vi "svc_Increment Histogram and Count.vi"(7 "counts in":T1, 10 "bin index":i32, 11 "histogram in":u64[](array[numeric])) -> (3 "histogram out":u64[](array[numeric]), 5 "counts out":T1)   [LabVIEW 2017]
uses:
  <vilib>/addons/_NISVFA/_Shared subVIs/Controls/svc_Histogram Counts.ctl
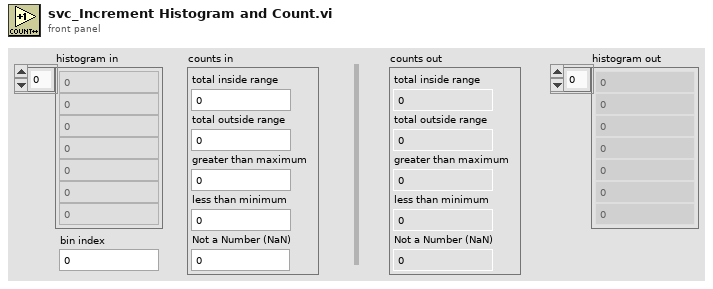
[diagram p1: front panel]
types:
  T1 = typedef "svc_Histogram Counts.ctl" = cluster{"total inside range":u64, "total outside range":u64, "greater than maximum":u64, "less than minimum":u64, "Not a Number (NaN)":u64}
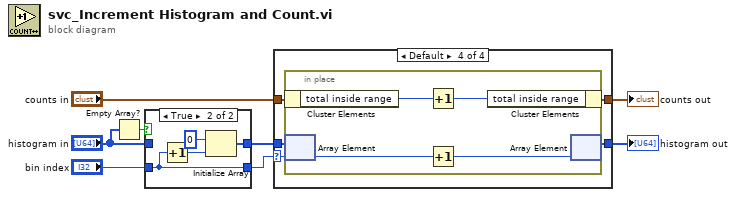
[diagram p0: block diagram]
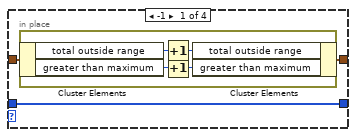
[diagram p3: hidden frame]
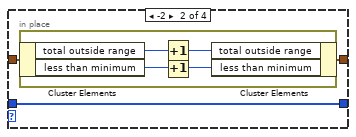
[diagram p4: hidden frame]
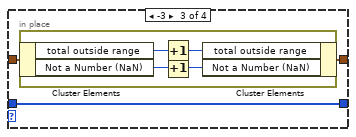
[diagram p5: hidden frame]
diagram:
  n1 = Empty Array?(array="histogram in") -> (empty?=w5:bool)
  n2 = case shown="True" w5 {
    tunnel: "histogram in" -> [w10 _]
    tunnel: "bin index" -> [w9 w11]
    tunnel: [w10 w12] -> w2
    tunnel: [w9 w11] -> w1
    frame False {
    }
    frame True {
      n3 = Increment(x=w11) -> (x+1=w14:i32)
      n4 = Initialize Array(u64 0 ("element"), w14) -> (w12:u64[])
    }
  }
  n5 = case shown="Default" w1 {
    selector: w1 -> [_ _ _ w39]
    tunnel: w2 -> [w15 w22 w31 w40]
    tunnel: [w16 w23 w29 w36] -> w6
    tunnel: "counts in" -> [w17 w24 w30 w37]
    tunnel: [w15 w22 w31 w38] -> w8
    frame -1 {
      n6 = in-place {
        n7 = in-place-cluster #1(w17) -> ("total outside range"=w21:u64, "greater than maximum"=w19:u64)
        n8 = Increment(x=w21) -> (x+1=w20:u64)
        n9 = Increment(x=w19) -> (x+1=w18:u64)
        n10 = in-place-cluster #1("total outside range"=w20, "greater than maximum"=w18) -> (w16:T1)
      }
    }
    frame -2 {
      n11 = in-place {
        n12 = in-place-cluster #2(w24) -> ("total outside range"=w28:u64, "less than minimum"=w26:u64)
        n13 = Increment(x=w28) -> (x+1=w27:u64)
        n14 = Increment(x=w26) -> (x+1=w25:u64)
        n15 = in-place-cluster #2("total outside range"=w27, "less than minimum"=w25) -> (w23:T1)
      }
    }
    frame -3 {
      n16 = in-place {
        n17 = in-place-cluster #3(w30) -> ("total outside range"=w35:u64, "Not a Number (NaN)"=w33:u64)
        n18 = Increment(x=w35) -> (x+1=w34:u64)
        n19 = Increment(x=w33) -> (x+1=w32:u64)
        n20 = in-place-cluster #3("total outside range"=w34, "Not a Number (NaN)"=w32) -> (w29:T1)
      }
    }
    frame Default {
      n21 = in-place {
        n22 = in-place-cluster #4(w37) -> ("total inside range"=w42:u64)
        n23 = in-place-array #5(w40, w39) -> (w44:u64)
        n24 = Increment(x=w42) -> (x+1=w41:u64)
        n25 = Increment(x=w44) -> (x+1=w43:u64)
        n26 = in-place-cluster #4("total inside range"=w41) -> (w36:T1)
        n27 = in-place-array #5(w43) -> (w38:u64[])  [unwired: 1 out]
      }
    }
  }
  "histogram out" <- w8
  "counts out" <- w6
